vi "errorCatcher.vi"(8 "error in (no error)":errorcluster, 11 "ExperimentRunner in":refnum<class "ExperimentRunner.lvclass">) -> (0 "error out":errorcluster, 3 "ExperimentRunner out":refnum<class "ExperimentRunner.lvclass">)   [LabVIEW 2009, in "Views.lvlib" / "ExperimentControl.lvlib" / "ExperimentRunner.lvclass"]
uses:
  ExperimentRunner.lvclass
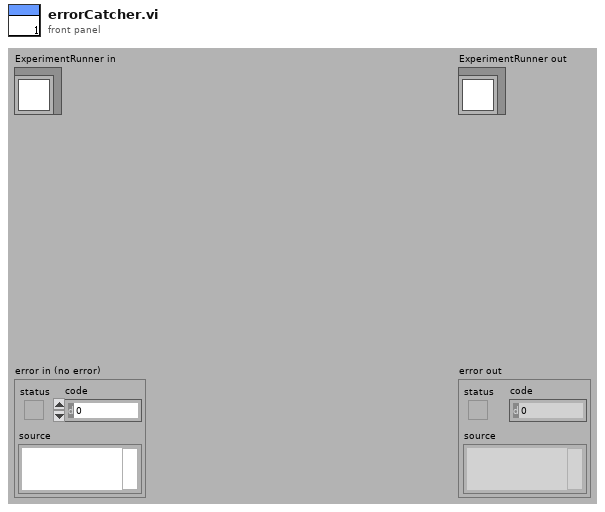
[diagram p1: front panel]
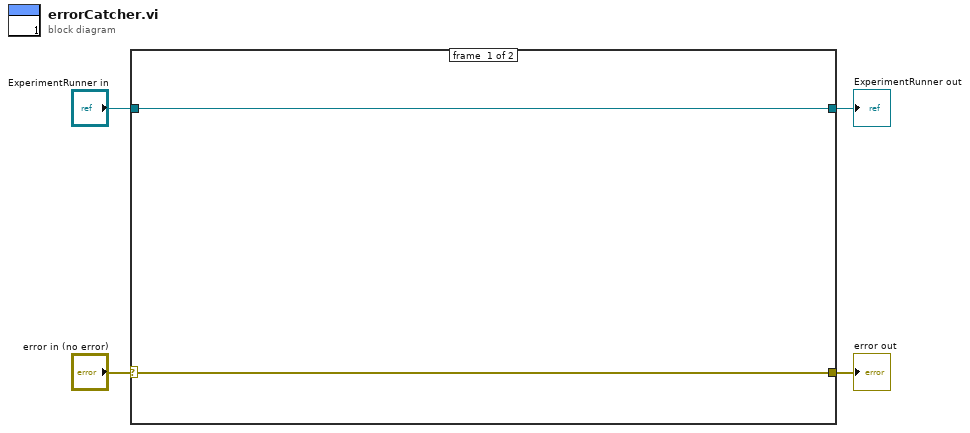
[diagram p0: block diagram]
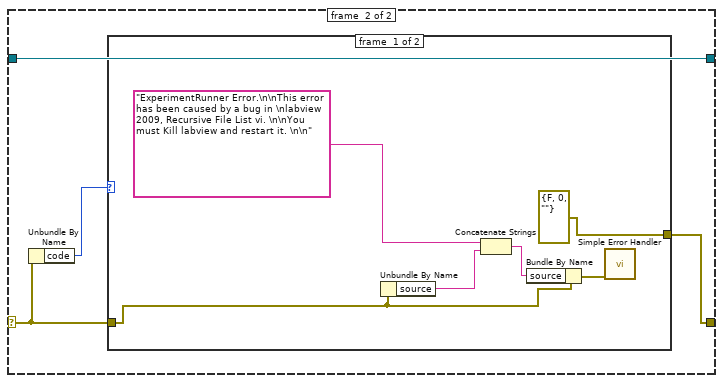
[diagram p2: hidden frame]
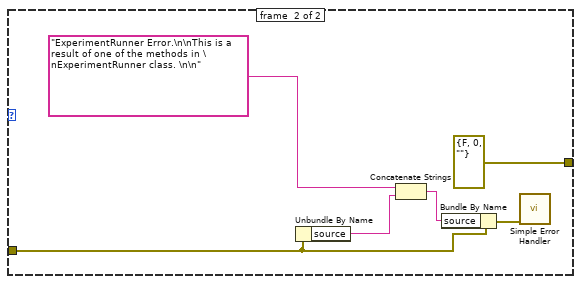
[diagram p3: hidden frame]
diagram:
  n1 = case shown="Error" "error in (no error)" {
    selector: "error in (no error)" -> [w5 w8]
    tunnel: [w5 w9] -> w3
    tunnel: [w6 w10] -> w1
    tunnel: "ExperimentRunner in" -> [w6 w10]
    frame #0 {
    }
    frame #1 {
      n2 = Unbundle By Name(w8) -> ("code"=w7:i32)
      n3 = case shown="7" w7 {
        tunnel: w8 -> [w11 w20]
        tunnel: [errorcluster {"status"=FALSE, "code"=0, "source"=""} ("error IO") errorcluster {"status"=FALSE, "code"=0, "source"=""} ("error IO")] -> w9
        frame #0 {
          n4 = Unbundle By Name(w11) -> ("source"=w15:string)
          n5 = Concatenate Strings("ExperimentRunner Error.\n\nThis error has been caused by a bug in \nlabview 2009, Recursive File List vi. \n\nYou must Kill labview and restart it. \n\n", w15) -> (w14:string)
          n6 = Bundle By Name(cluster=w11, "source"=w14) -> (w13:errorcluster)
          n7 = call <vilib>:"Simple Error Handler.vi"("error in (no error)"=w13) -> ()  [unwired: 4 in, 5 out]
        }
        frame #1 {
          n8 = Unbundle By Name(w20) -> ("source"=w21:string)
          n9 = Concatenate Strings("ExperimentRunner Error.\n\nThis is a result of one of the methods in \nExperimentRunner class. \n\n", w21) -> (w19:string)
          n10 = Bundle By Name(cluster=w20, "source"=w19) -> (w18:errorcluster)
          n11 = call <vilib>:"Simple Error Handler.vi"("error in (no error)"=w18) -> ()  [unwired: 4 in, 5 out]
        }
      }
    }
  }
  "error out" <- w3
  "ExperimentRunner out" <- w1
